vi "Search Complex Pair without Approximation.vi"(11 "Complex Numbers":cdb[](array[numeric])) -> (2 "Complex Pair Numbers":cdb[](array[numeric]), 3 "Pure Complex Numbers":cdb[](array[numeric]))   [LabVIEW 2017, in "NI_AALPro.lvlib"]
uses:
  <vilib>/Analysis/NI_AALPro.lvlib
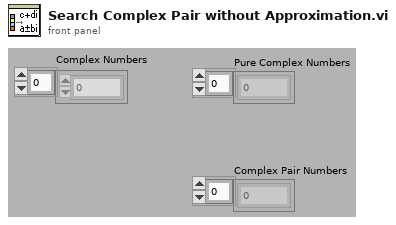
[diagram p1: front panel]
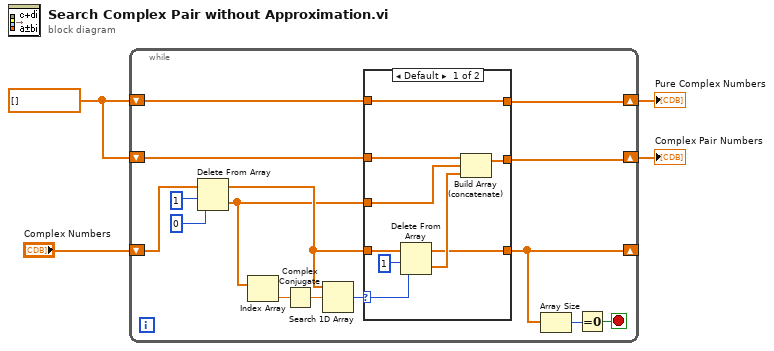
[diagram p0: block diagram]
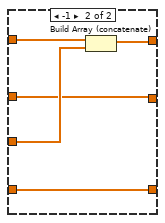
[diagram p2: hidden frame]
diagram:
  w3 = cdb[] [] ("CDB")
  n1 = while {
    shift-right: [w15] -> w2
    shift-left: w3 -> [w16]
    shift-right: [w12] -> _
    shift-left: "Complex Numbers" -> [w9]
    shift-right: [w13] -> w1
    shift-left: w3 -> [w14]
    stop <- w10 stop-if-true
    n2 = Delete From Array(array=w9, length=1, index=0) -> (deleted portion=w5:cdb[], array with subset deleted=w6:cdb[])
    n3 = Index Array(array=w5) -> (element=w19:cdb)  [unwired: 1 in]
    n4 = Complex Conjugate(1:w19) -> (0:w18:cdb)
    n5 = Search 1D Array(1D array=w6, element=w18) -> (index of element=w17:i32)  [unwired: 1 in]
    n6 = case shown="Default" w17 {
      selector: w17 -> [w26 _]
      tunnel: w16 -> [w25 w33]
      tunnel: [w25 w32] -> w15
      tunnel: w6 -> [w28 w29]
      tunnel: w14 -> [w24 w30]
      tunnel: [w23 w30] -> w13
      tunnel: [w20 w29] -> w12
      tunnel: w5 -> [w22 w31]
      frame Default {
        n7 = Delete From Array(array=w28, length=1, index=w26) -> (deleted portion=w21:cdb[], array with subset deleted=w20:cdb[])
        n8 = Build Array (concatenate)(w24, w22, w21) -> (w23:cdb[])
      }
      frame -1 {
        n9 = Build Array (concatenate)(w33, w31) -> (w32:cdb[])
      }
    }
    n10 = Array Size(array=w12) -> (size(s)=w11:i32)
    n11 = Equal To 0?(x=w11) -> (x = 0?=w10:bool)
  }
  "Pure Complex Numbers" <- w2
  "Complex Pair Numbers" <- w1
